vi "Robot Global Data.vi"() -> ()   [LabVIEW 2014]
doc: "This global VI can contain as many global variables as you need. Place a control on the panel, give it a good name. To read or write to it from a VI, drag the icon to the diagram of that VI. You can also drag from the project. Click on the node to change which global you access. You shouldn't have multiple locations writing to a global or it will cause a race-condition."
uses:
  <vilib>/Rock Robotics/WPI/Camera/WPI_CameraImageSize.ctl
  <vilib>/Rock Robotics/WPI/DriverStation/WPI_DriverStationRobotMode2.ctl
panel:
  in  "Elevator Safety Override":bool
  in  "Elevator Reset":bool
  in  "Feeder Lift Arms":bool
  in  "Feeder Drop Arms":bool
  in  "Feeder Lift Elevator":bool
  in  "Feeder Drop Elevator":bool
  in  "Feeder Roller":bool
  in  "Feeder Pickup":bool
  in  "Feeder Lift":bool
  in  "Feeder Drop":bool
  in  "Rotate Tote Right":bool
  in  "Rotate Tote Left":bool
  in  "Manual Clapper Out":bool
  in  "Manual Clapper In":bool
  in  "Manual Lower Arms":bool
  in  "Manual Raise Arms":bool
  in  "Motor Ramp":bool
  in  "Half Drive":bool
  in  "Clapper Out":bool
  in  "Elevator Modifier":bool
  in  "Elevator Pickup":bool
  in  "Elevator Down":bool
  in  "Elevator Up":bool
  in  "Right Joystick 2 X":dbl
  in  "Left Joystick 2 X":dbl
  in  "Right Joystick 2 Y":dbl
  in  "Left Joystick 2 Y":dbl
  in  "Clapper In":bool
  in  "Lower arms":bool
  in  "Raise arms":bool
  in  "Can Limit Switch":bool
  in  "Wiper":bool
  in  "Right Joystick X":dbl
  in  "Left Joystick X":dbl
  in  "Right Joystick Y":dbl
  in  "Left Joystick Y":dbl
  in  "Robot Mode":T1
  in  "image size":T2=enum."320x240"
  in  "Enable Vision":bool
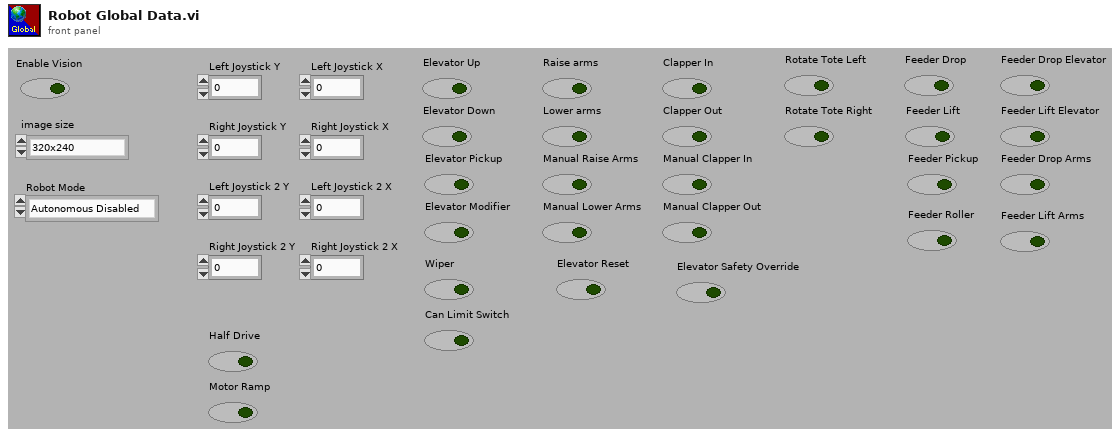
[diagram p1: front panel]
types:
  T1 = typedef "WPI_DriverStationRobotMode2.ctl" = enum16{"Autonomous Disabled", "Autonomous Enabled", "Teleop Disabled", "Teleop Enabled", "Disconnected", "Finish", "Test Disabled", "Test Enabled", "Emergency Stopped"}
  T2 = typedef "WPI_CameraImageSize.ctl" = enum16{"640x480", "320x240", "160x120", "Custom"}
diagram:
